vi "Send pretomo info.vi"(8 "error in (no error)":errorcluster, 11 "Tomo in":refnum<class "Tomo.lvclass">) -> (0 "error out":errorcluster, 3 "Tomo out":refnum<class "Tomo.lvclass">)   [LabVIEW 2012, in "Tomo.lvclass"]
uses:
  Tomo.lvclass
  <vilib>/Distrio/Murmex/Murmex/update_cluster.ctl
  Tomo.lvclass/Tomo.ctl
  <vilib>/Distrio/Murmex/Murmex/Murmex.lvclass
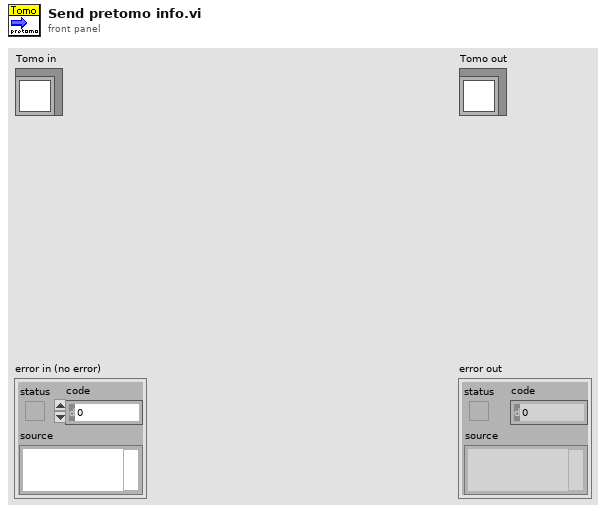
[diagram p1: front panel]
types:
  T1 = typedef "Murmex.lvlib/Murmex.lvclass/update_cluster.ctl" = cluster{"target ID":string, "key chains":string[], "values":variant[]}
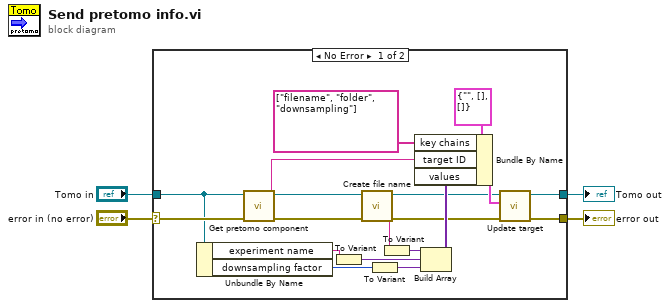
[diagram p0: block diagram]
diagram:
  n1 = case shown="No Error" "error in (no error)" {
    selector: "error in (no error)" -> [w13 w25]
    tunnel: [w15 w25] -> w3
    tunnel: [w16 w24] -> w1
    tunnel: "Tomo in" -> [w10 w24]
    frame No Error {
      n2 = Unbundle By Name(w10) -> ("experiment name"=w6:string, "downsampling factor"=w9:u32)
      n3 = call-dynamic "Get pretomo component.vi"("error in (no error)"=w13, "Tomo in"=w10) -> ("error out"=w14:errorcluster, "pretomo camera component"=w8:string, "Tomo out"=w18:refnum<class "Tomo.lvclass">)  [unwired: 7 in]
      n4 = To Variant(anything=w6) -> (Variant=w5:variant)
      n5 = call-dynamic "Create file name.vi"("error in (no error)"=w14, "Tomo in"=w18) -> ("error out"=w12:errorcluster, "filename"=w11:string, "Tomo out"=w17:refnum<class "Tomo.lvclass">)  [unwired: 7 in]
      n6 = To Variant(anything=w9) -> (Variant=w7:variant)
      n7 = To Variant(anything=w11) -> (Variant=w20:variant)
      n8 = Build Array(w20, w5, w7) -> (w22:variant[])
      n9 = Bundle By Name(cluster=T1 {"target ID"="", "key chains"=[], "values"=[]} ("update cluster"), "key chains"=string[] ["filename", "folder", "downsampling"], "target ID"=w8, "values"=w22) -> (w23:T1)
      n10 = call <vilib>:"Update target.vi"("error in (no error)"=w12, "update cluster"=w23, "MurmexBase in"=w17) -> ("error out"=w15:errorcluster, "MurmexBase out"=w16:refnum<class "Tomo.lvclass">)  [unwired: 7 in]
    }
    frame Error {
    }
  }
  "error out" <- w3
  "Tomo out" <- w1
